vi "Populate Run-Time Menu.vi"(8 "error in (no error)":errorcluster, 10 "Menu in":refnum<k9>, 11 "Execution UI In":refnum<class "Execution UI.lvclass">) -> (0 "error out":errorcluster, 3 "Execution UI Out":refnum<class "Execution UI.lvclass">)   [LabVIEW 2020, in "Execution UI.lvclass"]
uses:
  Execution UI.lvclass
  Execution UI.lvclass/Execution UI.ctl
  Framework/Report Plugin/Report Plugin.lvclass
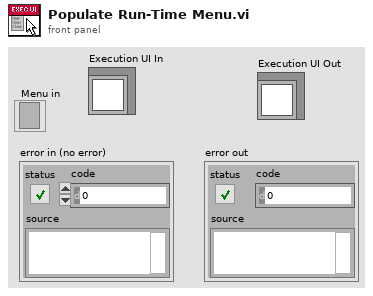
[diagram p1: front panel]
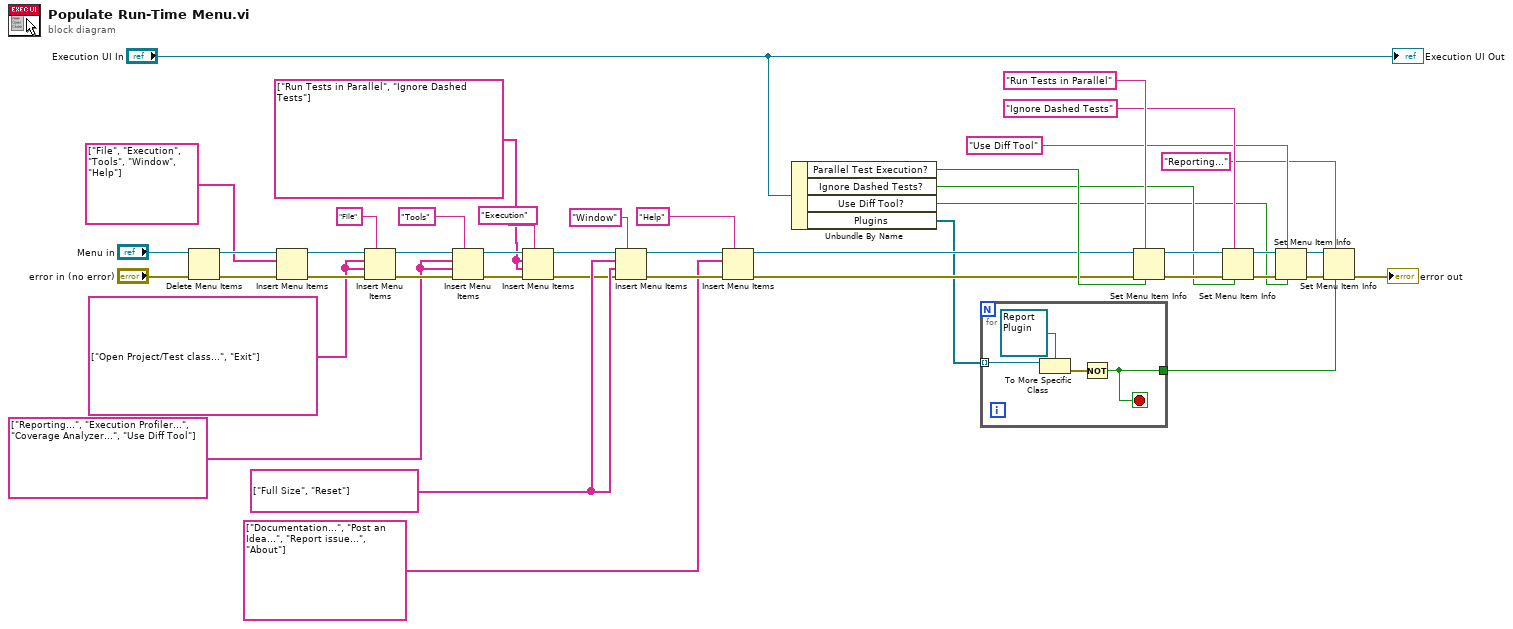
[diagram p0: block diagram]
diagram:
  w7 = string[] ["Run Tests in Parallel", "Ignore Dashed Tests"] ("item names")
  w27 = string[] ["Full Size", "Reset"] ("item names")
  w28 = string[] ["Reporting...", "Execution Profiler...", "Coverage Analyzer...", "Use Diff Tool"] ("item names")
  w26 = string[] ["Open Project/Test class...", "Exit"] ("item names")
  n1 = Delete Menu Items(6:"error in (no error)", 9:"Menu in") -> (0:w41:errorcluster, 3:w43:refnum<k9>)  [unwired: 2 in]
  n2 = Insert Menu Items(6:w41, 8:string[] ["File", "Execution", "Tools", "Window", "Help"] ("item names"), 9:w43) -> (0:w38:errorcluster, 3:w39:refnum<k9>)  [unwired: 3 in, 1 out]
  n3 = Insert Menu Items(5:"File" ("menu tag"), 6:w38, 7:w26, 8:w26, 9:w39) -> (0:w35:errorcluster, 3:w34:refnum<k9>)  [unwired: 1 in, 1 out]
  n4 = Insert Menu Items(5:"Tools", 6:w35, 7:w28, 8:w28, 9:w34) -> (0:w12:errorcluster, 3:w9:refnum<k9>)  [unwired: 1 in, 1 out]
  n5 = Insert Menu Items(5:"Execution", 6:w12, 7:w7, 8:w7, 9:w9) -> (0:w11:errorcluster, 3:w10:refnum<k9>)  [unwired: 1 in, 1 out]
  n6 = Insert Menu Items(5:"Window", 6:w11, 7:w27, 8:w27, 9:w10) -> (0:w36:errorcluster, 3:w33:refnum<k9>)  [unwired: 1 in, 1 out]
  n7 = Insert Menu Items(5:"Help", 6:w36, 8:string[] ["Documentation...", "Post an Idea...", "Report issue...", "About"] ("item names"), 9:w33) -> (0:w21:errorcluster, 3:w23:refnum<k9>)  [unwired: 2 in, 1 out]
  n8 = Unbundle By Name("Execution UI In") -> ("Parallel Test Execution?"=w24:bool, "Ignore Dashed Tests?"=w17:bool, "Use Diff Tool?"=w13:bool, "Plugins"=w2:refnum<class "Plugin.lvclass">[])
  n9 = for {
    tunnel: w2 -> [w48] mode=indexing
    tunnel: [w45] -> w1
    stop <- w45 stop-if-true
    n10 = To More Specific Class(target class=refnum<class "Report Plugin.lvclass"> refnum ("Reports.lvlib:Report Interface.lvclass"), reference=w48) -> (error out=w47:errorcluster)  [unwired: 1 in, 1 out]
    n11 = Not(x=w47) -> (.not. x?=w45:bool)
  }
  n12 = Set Menu Item Info(6:w24, 7:"Run Tests in Parallel", 8:w21, 11:w23) -> (0:w19:errorcluster, 3:w20:refnum<k9>)  [unwired: 3 in]
  n13 = Set Menu Item Info(6:w17, 7:"Ignore Dashed Tests", 8:w19, 11:w20) -> (0:w16:errorcluster, 3:w15:refnum<k9>)  [unwired: 3 in]
  n14 = Set Menu Item Info(6:w13, 7:"Use Diff Tool", 8:w16, 11:w15) -> (0:w5:errorcluster, 3:w6:refnum<k9>)  [unwired: 3 in]
  n15 = Set Menu Item Info(6:w1, 7:"Reporting...", 8:w5, 11:w6) -> (0:→"error out":errorcluster)  [unwired: 3 in, 1 out]
  "Execution UI Out" <- "Execution UI In"
